vi "4Pi OIA - Get Image.vi"(0 "Camera Notifier Name":string, 2 "Alignment Data":T1={"Action"=enum."Start Alignment", "ROI Selection"=enum."Full Image", "Method"=enum."2D Gaussian Fit", "Frame Accums."=0, "Camera Px. Size (µm)"=0.0, "Image Ref"=refnum}) -> (8 "Image Out":u16[][](array[numeric]))   [LabVIEW 2016]
uses:
  4Pi OIA - Controls/4Pi OIA - Notifier Type.ctl
  4Pi OIA - Controls/4Pi OIA - Actions.ctl
  4Pi OIA - Controls/4Pi OIA - ROI Selection.ctl
  4Pi OIA - Controls/4Pi OIA - Method.ctl
  <vilib>/vision/Image Controls.llb/IMAQ Image.ctl
  Device Library/Cameras/Hamamatsu/Orca Flash/Orca Flash Controls/Orca Flash Actions.ctl
  Device Library/Cameras/Camera Controls/Camera IMAQ Key Info.ctl
  Display Module/Display Module Custom Controls/ROI Descriptor.ctl
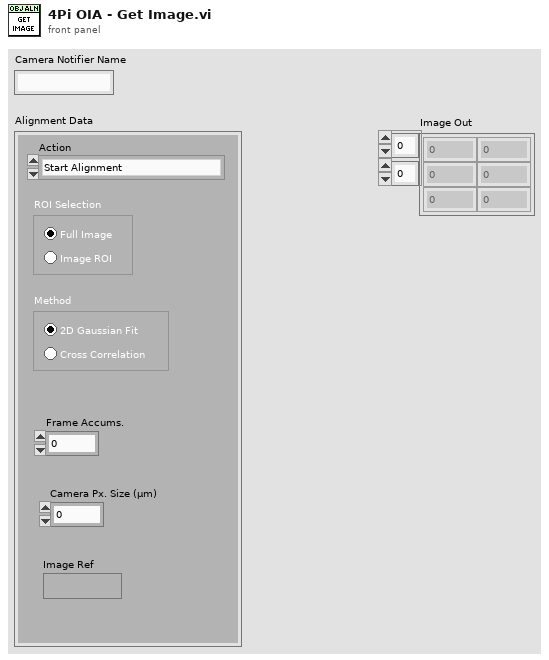
[diagram p1: front panel]
types:
  T1 = typedef "4Pi OIA - Notifier Type.ctl" = cluster{"Action":T2, "ROI Selection":T3, "Method":T4, "Frame Accums.":u16, "Camera Px. Size (µm)":dbl, "Image Ref":T5}
  T2 = typedef "4Pi OIA - Actions.ctl" = enum16{"Idle", "Start Alignment", "Get Upper Image", "Get Lower Image", "Get Shift", "Move OBJ", "Quit"}
  T3 = typedef "4Pi OIA - ROI Selection.ctl" = enum32{"Full Image", "ROI"}
  T4 = typedef "4Pi OIA - Method.ctl" = enum32{"2D Gaussian Fit", "Cross Correlation"}
  T5 = typedef "IMAQ Image.ctl" = refnum<image>
  T6 = typedef "Orca Flash Actions.ctl" = enum16{"IDLE", "PREVIEW", "RECORD", "Record Settings", "SETPARAM", "GETPARAM", "SETROI", "GETROI", "PROGRESSIVE MODE", "AREA MODE", "STATUS", "QUIT"}
  T7 = typedef "ROI Descriptor.ctl" = cluster{"Global Rectangle":i32[], "Contours":cluster{"Contour Type":u32, "ROI Type":u32, "Points":i32[]}[]}
  T8 = typedef "Camera IMAQ Key Info.ctl" = cluster{"Frame":u32, "Sensor Height":i32, "Sensor Width":i32, "ROI Height":i32, "ROI Width":i32, "ROI Enable?":bool, "Bit per Pixel":u8}
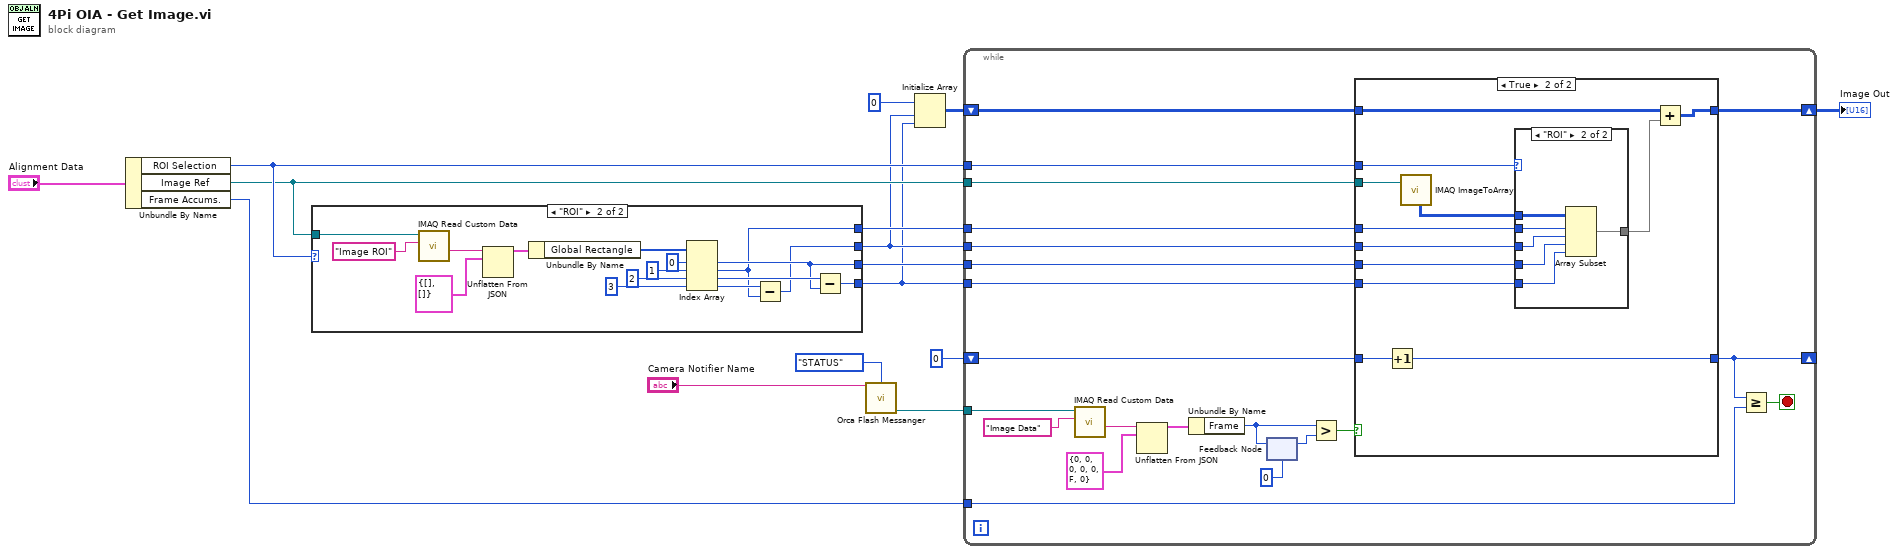
[diagram p0: block diagram]
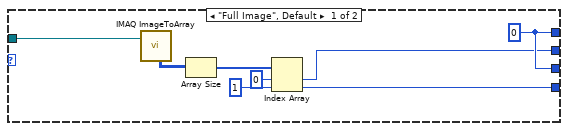
[diagram p2: hidden frame]
diagram:
  n1 = Unbundle By Name("Alignment Data") -> ("ROI Selection"=w8:T3, "Image Ref"=w7:T5, "Frame Accums."=w2:u16)
  n2 = case shown="\"ROI\"" w8 {
    tunnel: w7 -> [w22 w30]
    tunnel: [w23 w27] -> w5
    tunnel: [w16 w26] -> w3
    tunnel: [w23 w25] -> w6
    tunnel: [w17 w24] -> w4
    frame "Full Image", Default {
      w23 = 0
      n3 = call "IMAQ ImageToArray"("Image"=w22) -> ("Image Pixels (U16)"=w21:u16[][])  [unwired: 3 in, 4 out]
      n4 = Array Size(array=w21) -> (size(s)=w20:i32[])
      n5 = Index Array(array=w20, index #1=0 ("index"), index #2=1 ("index")) -> (element #1=w17:i32, element #2=w16:i32)
    }
    frame "ROI" {
      n6 = call "IMAQ Read Custom Data"("Key"="Image ROI", "Image"=w30) -> ("Custom Data Out"=w38:string)  [unwired: 7 in, 2 out]
      n7 = Unflatten From JSON(JSON string=w38, type and defaults=T7 {"Global Rectangle"=[], "Contours"=[]} ("Image ROI Descriptor")) -> (value=w36:T7)  [unwired: 5 in, 1 out]
      n8 = Unbundle By Name(w36) -> ("Global Rectangle"=w35:i32[])
      n9 = Index Array(array=w35, index #1=0 ("index"), index #2=1 ("index"), index #3=2 ("index"), index #4=3 ("index")) -> (element #1=w27:i32, element #2=w25:i32, element #3=w28:i32, element #4=w29:i32)
      n10 = Subtract(x=w29, y=w25) -> (x-y=w24:i32)
      n11 = Subtract(x=w28, y=w27) -> (x-y=w26:i32)
    }
  }
  n12 = call "Orca Flash Messanger.vi"("Notifier Name"="Camera Notifier Name", "Camera Actions"=Orca_Flash_Actions."STATUS") -> ("Image Ref"=w12:T5)  [unwired: 9 in, 4 out]
  n13 = Initialize Array(u16 0, w4, w3) -> (w10:u16[][])
  n14 = while {
    tunnel: w12 -> [w56]
    shift-right: [w50] -> _
    shift-left: u16 0 -> [w51]
    tunnel: w8 -> [w48]
    tunnel: w7 -> [w47]
    shift-right: [w41] -> w1
    shift-left: w10 -> [w42]
    tunnel: w6 -> [w46]
    tunnel: w4 -> [w45]
    tunnel: w5 -> [w44]
    tunnel: w3 -> [w43]
    tunnel: w2 -> [w40]
    stop <- w49 stop-if-true
    n15 = call "IMAQ Read Custom Data"("Key"="Image Data", "Image"=w56) -> ("Custom Data Out"=w58:string)  [unwired: 7 in, 2 out]
    n16 = Unflatten From JSON(JSON string=w58, type and defaults=T8 {"Frame"=0, "Sensor Height"=0, "Sensor Width"=0, "ROI Height"=0, "ROI Width"=0, "ROI Enable?"=FALSE, "Bit per Pixel"=0} ("Camera IMAQ Key Info")) -> (value=w60:T8)  [unwired: 5 in, 1 out]
    n17 = Unbundle By Name(w60) -> ("Frame"=w53:u32)
    n18 = feedback #1(u32 0 ("Frame")) -> (w55:u32)
    n19 = feedback-in #1(w53) -> ()
    n20 = Greater?(x=w53, y=w55) -> (0:w52:bool)
    n21 = case shown="True" w52 {
      tunnel: w51 -> [w62 w74]
      tunnel: [w62 w73] -> w50
      tunnel: w48 -> [_ w72]
      tunnel: w47 -> [_ w71]
      tunnel: w46 -> [_ w69]
      tunnel: w45 -> [_ w68]
      tunnel: w44 -> [_ w67]
      tunnel: w43 -> [_ w66]
      tunnel: w42 -> [w61 w65]
      tunnel: [w61 w63] -> w41
      frame False {
      }
      frame True {
        n22 = Increment(x=w74) -> (x+1=w73:u16)
        n23 = call "IMAQ ImageToArray"("Image"=w71) -> ("Image Pixels (U16)"=w70:u16[][])  [unwired: 3 in, 4 out]
        n24 = case shown="\"ROI\"" w72 {
          tunnel: w70 -> [w75 w81]
          tunnel: w69 -> [_ w80]
          tunnel: w68 -> [_ w79]
          tunnel: w67 -> [_ w78]
          tunnel: w66 -> [_ w77]
          tunnel: [w75 w76] -> w64
          frame "Full Image", Default {
          }
          frame "ROI" {
            n25 = Array Subset(array=w81, index (row)=w80, length (row)=w79, index (col)=w78, length (col)=w77) -> (w76:u16[][])
          }
        }
        n26 = Add(x=w65, y=w64) -> (x+y=w63:u16[][])
      }
    }
    n27 = Greater Or Equal?(x=w50, y=w40) -> (x >= y?=w49:bool)
  }
  "Image Out" <- w1
